vi "Git-JSON array string to 2D string array.vi"(8 "error in (no error)":errorcluster, 11 "Response body":string) -> (0 "error out":errorcluster, 3 "Array":string[][][](array[string]))   [LabVIEW 2020]
uses:
  <vilib>/JDP Science/JSONtext/JSONtext.lvlib
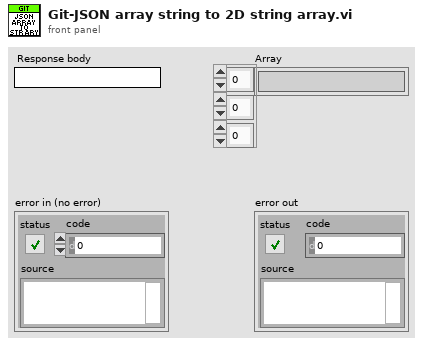
[diagram p1: front panel]
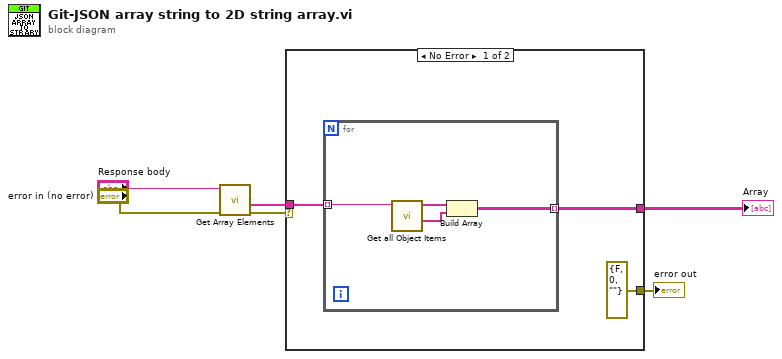
[diagram p0: block diagram]
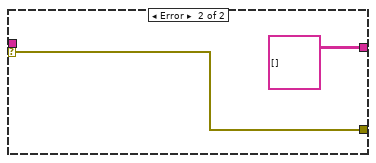
[diagram p2: hidden frame]
diagram:
  n1 = call <vilib>:"Get Array Elements.vi"("error in (no error)"="error in (no error)", "JSON"="Response body") -> ("error out"=w1:errorcluster, "<JSON>"=w2:string[])  [unwired: 7 in, 1 out]
  n2 = case shown="No Error" w1 {
    selector: w1 -> [_ w14]
    tunnel: w2 -> [w9 _]
    tunnel: [w8 string[][][] []] -> w5
    tunnel: [errorcluster {"status"=FALSE, "code"=0, "source"=""} ("error IO") w14] -> w3
    frame No Error {
      n3 = for {
        tunnel: w9 -> [w13] mode=indexing
        tunnel: [w10] -> w8 mode=indexing
        n4 = call <vilib>:"Get all Object Items.vi"("JSON"=w13) -> ("<JSON>"=w11:string[], "Item Names"=w12:string[])  [unwired: 7 in, 2 out]
        n5 = Build Array(w12, w11) -> (w10:string[][])
      }
    }
    frame Error {
    }
  }
  "error out" <- w3
  "Array" <- w5
